vi "PV HLT5xx Relay mode.vi"(6 "set Relay 2":u16(ring)=4 items=["off", "Start (V2 opened)", "Stop (V6 opened)", "Start / Stop", "measure", "threshold leakrate", "on", "Warn limit leakrate", "threshold pressure"], 7 "Adress of unit":u16=1 min=1 max=999 step=1, 8 "error in (no error)":errorcluster, 9 "set Relay 1":u16(ring)=3 items=["off", "Start (V2 opened)", "Stop (V6 opened)", "Start / Stop", "measure", "threshold leakrate", "on", "Warn limit leakrate", "threshold pressure"], 10 "Parameter\nread only<->describe":bool, 11 "VISA session":refnum<visa-resource-name>) -> (0 "error out":errorcluster, 1 "Relay 1 out":u16(ring)=3 items=["off", "Start (V2 opened)", "Stop (V6 opened)", "Start / Stop", "measure", "threshold leakrate", "on", "Warn limit leakrate", "threshold pressure"], 2 "response (data)":string, 3 "dup VISA session":refnum<visa-resource-name>, 4 "Relay 2 out":u16(ring)=4 items=["off", "Start (V2 opened)", "Stop (V6 opened)", "Start / Stop", "measure", "threshold leakrate", "on", "Warn limit leakrate", "threshold pressure"])   [LabVIEW 2021, in "Pfeiffer Vacuum.lvlib"]
doc: "This VI allows you to set or check the \"Relay Mode (Para 684)\" on the SmartTest (HLT5xx)."
uses:
  <instrlib>/Pfeiffer Vacuum/Pfeiffer Vacuum.lvlib
panel:
  # "Relay mode"
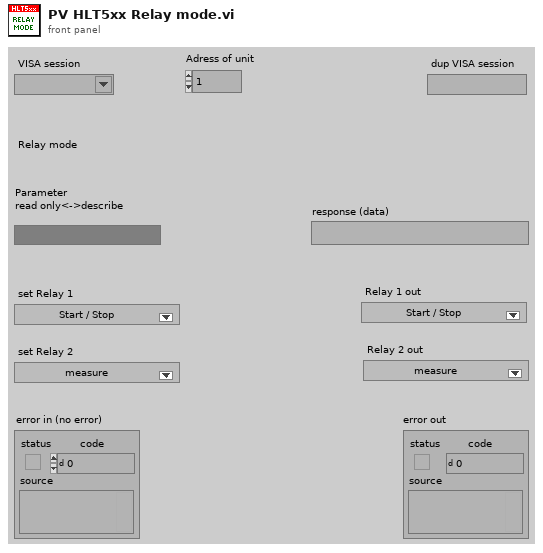
[diagram p1: front panel]
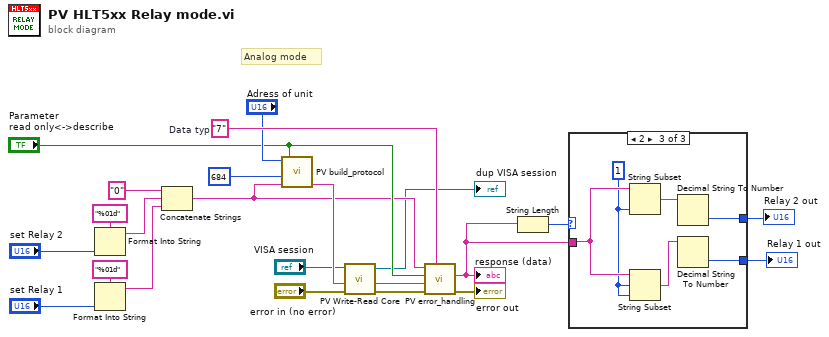
[diagram p0: block diagram]
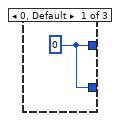
[diagram p2: hidden frame]
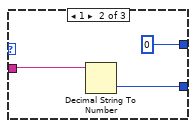
[diagram p3: hidden frame]
diagram:
  w19 = "7"  # Data typ
  # "Analog mode"
  n1 = Format Into String(format string="%01d" ("Format-String"), "set Relay 2") -> (resulting string=w10:string)  [unwired: 2 in, 1 out]
  n2 = Format Into String(format string="%01d" ("Format-String"), "set Relay 1") -> (resulting string=w9:string)  [unwired: 2 in, 1 out]
  n3 = Concatenate Strings("0" ("Resultierender String"), w10, w9) -> (w8:string)
  n4 = call <instrlib>:"PV build_protocol.vi"("Data"=w8, "Parameter-number"=u16 684, "parameter\nread<->describe"="Parameter\nread only<->describe", "Adress"="Adress of unit") -> ("output"=w22:string)  [unwired: 3 in]
  n5 = call <instrlib>:"PV Write-Read Core.vi"("error in"="error in (no error)", "Write data in"=w22, "VISA session"="VISA session") -> ("error out"=w20:errorcluster, "response (data) out"=w21:string, "dup VISA session"=→"dup VISA session":refnum<visa-resource-name>)  [unwired: 2 in]
  n6 = call <instrlib>:"PV error_handling.vi"("Data Typ in"=w19, "error in"=w20, "response (data) in"=w21, "Parameter\nread only<->describe"="Parameter\nread only<->describe", "data in"=w8) -> ("error out"=→"error out":errorcluster, "Data out"=w5:string)  [unwired: 4 in, 1 out]
  "response (data)" <- w5
  n7 = String Length(string=w5) -> (length=w6:i32)
  n8 = case shown="2" w6 {
    tunnel: w5 -> [_ w27 w31]
    tunnel: [w24 0 w32] -> w3
    tunnel: [w24 w25 w33] -> w4
    frame 0, Default {
      w24 = 0
    }
    frame 1 {
      n9 = Decimal String To Number(string=w27) -> (number=w25:i32)  [unwired: 2 in, 1 out]
    }
    frame 2 {
      w28 = 1
      n10 = String Subset(string=w31, length (rest)=w28) -> (substring=w30:string)  [unwired: 1 in]
      n11 = String Subset(string=w31, offset (0)=w28, length (rest)=w28) -> (substring=w29:string)
      n12 = Decimal String To Number(string=w30) -> (number=w32:i32)  [unwired: 2 in, 1 out]
      n13 = Decimal String To Number(string=w29) -> (number=w33:i32)  [unwired: 2 in, 1 out]
    }
  }
  "Relay 1 out" <- w4
  "Relay 2 out" <- w3
